vi "CLSUIP_GetNestedControlNames.vi"(8 "error in (no error)":errorcluster, 11 "Ctl Refnum":refnum<vi>) -> (0 "error out":errorcluster, 2 "Element names":string[](array[string]), 3 "Ctl Refnum out":refnum<vi>)   [LabVIEW 2021, in "MemberVICreation.lvlib"]
uses:
  <resource>/Framework/Providers/LVClassLibrary/NewAccessors/MemberVICreation.lvlib
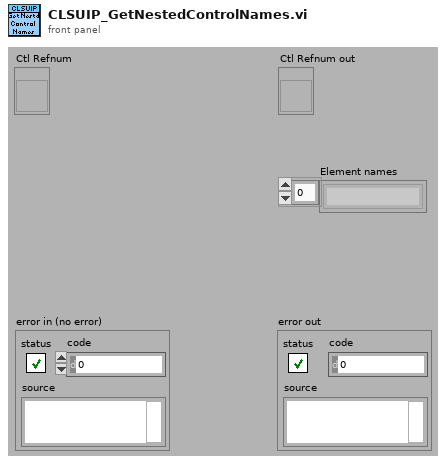
[diagram p1: front panel]
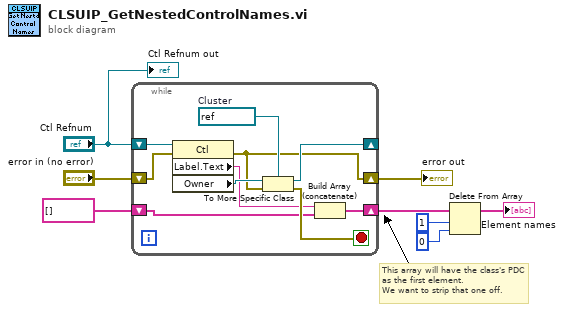
[diagram p0: block diagram]
diagram:
  # "This array will have the class's PDC as the first element.\nWe want to strip that one off."
  n1 = while {
    shift-right: [w10] -> w4
    shift-left: string[] [] ("Element names") -> [w12]
    shift-right: [w14] -> _
    shift-left: "Ctl Refnum" -> [w18]
    shift-right: [w9] -> w5
    shift-left: "error in (no error)" -> [w17]
    stop <- w13 stop-if-true
    w16 = refnum<vi> refnum  # Cluster
    n2 = property class="Ctl"(reference=w18, error in=w17) -> (error out=w9:errorcluster, "Label.Text"=w11:string, "Owner"=w15:refnum<vi>)  [unwired: 1 out]
    n3 = To More Specific Class(target class=w16, reference=w15, error in=w9) -> (specific class reference=w14:refnum<vi>, error out=w13:errorcluster)
    n4 = Build Array (concatenate)(w11, w12) -> (w10:string[])
  }
  "error out" <- w5
  n5 = Delete From Array(array=w4, length=1, index=0) -> (array with subset deleted=→"Element names":string[])  [unwired: 1 out]
  "Ctl Refnum out" <- "Ctl Refnum"
